vi "PH_uOPA_DelayController.ProcEvents.vi"(0 "i ref in":refnum<vi>, 5 "error in":errorcluster) -> (14 "i ref out":refnum<vi>, 19 "error out":errorcluster)   [LabVIEW 2014, in "PH_uOPA_DelayController.lvlib"]
doc: "This method is used to define the events the object will listen to. Add your own events here."
uses:
  PH_uOPA_DelayController.lvlib
  CS_Core/BaseProcess/BaseProcess.event definition.ctl
  CS_Core/CAEObj/CAEObj.event definition.ctl
  CS_Core/BaseProcess/BaseProcess.descriptor string definition.ctl
  CS_Core/BaseProcess/BaseProcess.lvlib
  CS_Core/CAEObj/CAEObj.lvlib
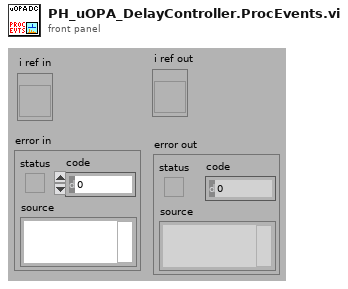
[diagram p1: front panel]
types:
  T1 = typedef "BaseProcess.lvlib/BaseProcess.event definition.ctl" = cluster{"CAEEvtDef":T2, "Data Descriptor":T3}
  T2 = typedef "CAEObj.lvlib/CAEObj.event definition.ctl" = cluster{"URL":string, "enable":bool, "ignoreResID":bool}
  T3 = typedef "BaseProcess.lvlib/BaseProcess.descriptor string definition.ctl" = string
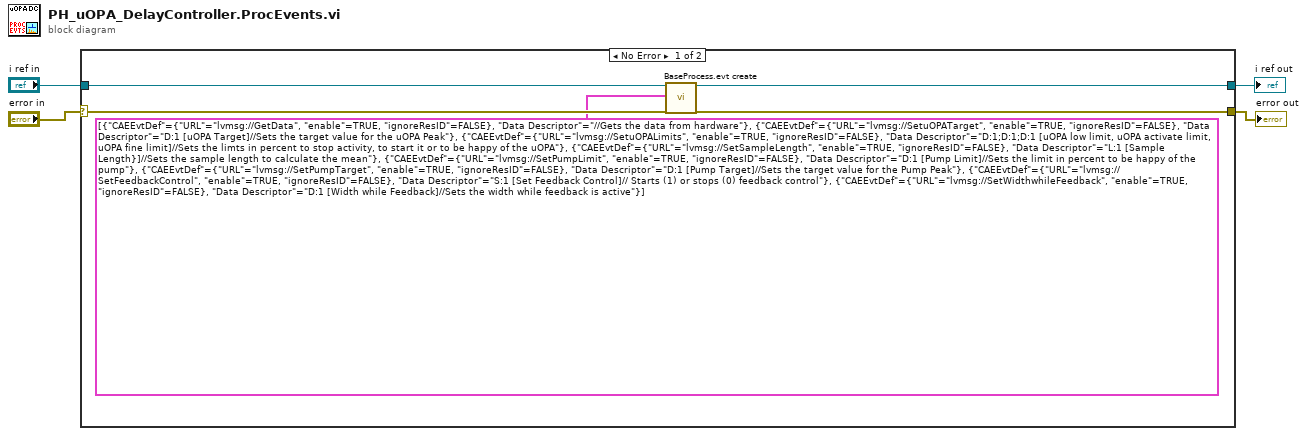
[diagram p0: block diagram]
diagram:
  n1 = case shown="No Error" "error in" {
    selector: "error in" -> [w7 w10]
    tunnel: "i ref in" -> [w6 w11]
    tunnel: [w9 w11] -> w3
    tunnel: [w8 w10] -> w2
    frame No Error {
      n2 = call "BaseProcess.evt create.vi"("i ref in"=w6, "newEvents"=T1[] [{"CAEEvtDef"={"URL"="lvmsg://GetData", "enable"=TRUE, "ignoreResID"=FALSE}, "Data Descriptor"="//Gets the data from hardware"}, {"CAEEvtDef"={"URL"="lvmsg://SetuOPATarget", "enable"=TRUE, "ignoreResID"=FALSE}, "Data Descriptor"="D:1 [uOPA Target]//Sets the target value for the uOPA Peak"}, {"CAEEvtDef"={"URL"="lvmsg://SetuOPALimits", "enable"=TRUE, "ignoreResID"=FALSE}, "Data Descriptor"="D:1;D:1;D:1 [uOPA low limit, uOPA activate limit, uOPA fine limit]//Sets the limts in percent to stop activity, to start it or to be happy of the uOPA"}, {"CAEEvtDef"={"URL"="lvmsg://SetSampleLength", "enable"=TRUE, "ignoreResID"=FALSE}, "Data Descriptor"="L:1 [Sample Length}]//Sets the sample length to calculate the mean"}, {"CAEEvtDef"={"URL"="lvmsg://SetPumpLimit", "enable"=TRUE, "ignoreResID"=FALSE}, "Data Descriptor"="D:1 [Pump Limit]//Sets the limit in percent to be happy of the pump"}, {"CAEEvtDef"={"URL"="lvmsg://SetPumpTarget", "enable"=TRUE, "ignoreResID"=FALSE}, "Data Descriptor"="D:1 [Pump Target]//Sets the target value for the Pump Peak"}, {"CAEEvtDef"={"URL"="lvmsg://SetFeedbackControl", "enable"=TRUE, "ignoreResID"=FALSE}, "Data Descriptor"="S:1 [Set Feedback Control]// Starts (1) or stops (0) feedback control"}, {"CAEEvtDef"={"URL"="lvmsg://SetWidthwhileFeedback", "enable"=TRUE, "ignoreResID"=FALSE}, "Data Descriptor"="D:1 [Width while Feedback]//Sets the width while feedback is active"}] ("new events"), "error in (no error)"=w7) -> ("i ref out"=w9:refnum<vi>, "error out"=w8:errorcluster)  [unwired: 13 in, 2 out]
    }
    frame Error {
    }
  }
  "i ref out" <- w3
  "error out" <- w2
